vi "GetTime_Video.vi"(8 "error in (no error)":errorcluster, 11 "VLC Variables In":T1) -> (0 "error out":errorcluster, 1 "Player Time":i32, 3 "VLC Variables Out":T1)   [LabVIEW 2012]
doc: "Get the elapsed time since the video began."
uses:
  Controls-Webcam/VLC Var.ctl
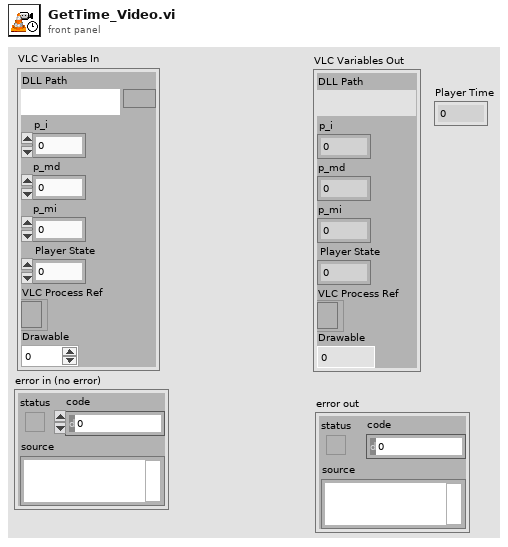
[diagram p1: front panel]
types:
  T1 = typedef "VLC Var.ctl" = cluster{"DLL Path":path, "p_i":i32, "p_md":i32, "p_mi":i32, "Player State":i32, "VLC Process Ref":refnum<k24>, "Drawable":i32}
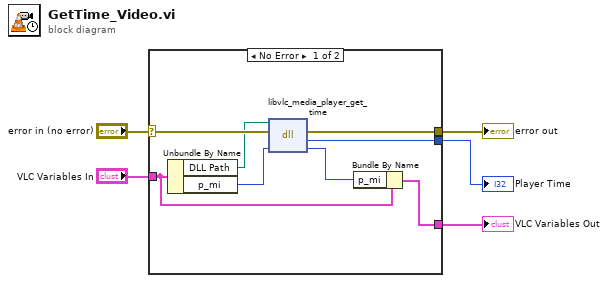
[diagram p0: block diagram]
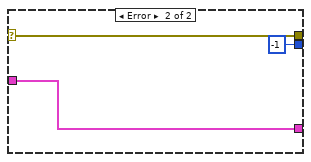
[diagram p2: hidden frame]
diagram:
  n1 = case shown="No Error" "error in (no error)" {
    selector: "error in (no error)" -> [w8 w16]
    tunnel: [w13 w16] -> w5
    tunnel: [w12 -1 ("return type")] -> w4
    tunnel: [w10 w15] -> w3
    tunnel: "VLC Variables In" -> [w6 w15]
    frame No Error {
      n2 = Unbundle By Name(w6) -> ("DLL Path"=w7:path, "p_mi"=w11:i32)
      n3 = dll-call lib="C:/Program Files/VideoLAN/VLC/libvlc.dll" fn="libvlc_media_player_get_time"(path in=w7, error in=w8, "p_mi"=w11) -> (error out=w13:errorcluster, "return type"=w12:i32, "p_mi"=w9:i32)  [unwired: 1 in, 1 out]
      n4 = Bundle By Name(cluster=w6, "p_mi"=w9) -> (w10:T1)
    }
    frame Error {
    }
  }
  "error out" <- w5
  "Player Time" <- w4
  "VLC Variables Out" <- w3
